vi "Manager.vi"   [LabVIEW 2021, in "Plugin Manager.lvclass"]
uses:
  Plugin Manager.lvclass
  CIFUtilities/CIFClocks/Time Conversion/LabVIEW Time to UTC Time.vi
  CIFCore/Common/Utilities/Add Error.vi
  CIFCore/Common/Utilities/Append Error Location.vi
  CIFUtilities/CIFClocks/CIFClocks.lvlib
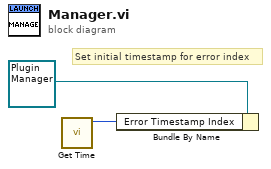
[diagram p0: block diagram]
diagram:
  # "Set initial timestamp for error index"
  n1 = call "Get Time.vi"() -> ("Time (ns)"=w1:u64)  [unwired: 9 in, 2 out]
  n2 = Bundle By Name(cluster=refnum<class "Plugin Manager.lvclass"> refnum ("Plugin Manager.lvclass"), "Error Timestamp Index"=w1) -> ()  [unwired: 1 out]
